vi "DeferPanelUpdate.vi"(8 "VI in":refnum<vi>, 10 "defer panel updates":bool, 11 "error in (no error)":errorcluster) -> (0 "VI out":refnum<vi>, 3 "error out":errorcluster)   [LabVIEW 2013]
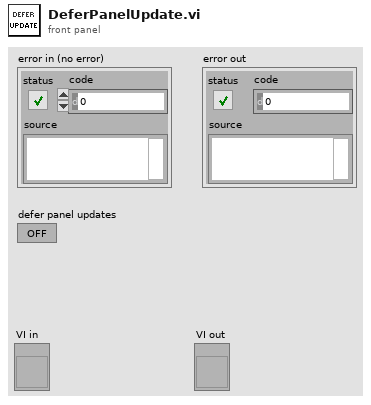
[diagram p1: front panel]
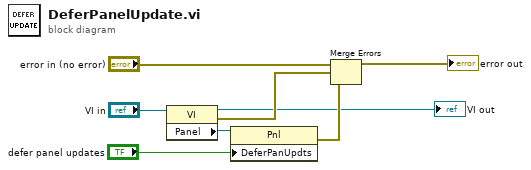
[diagram p0: block diagram]
diagram:
  n1 = property class="VI"(reference="VI in") -> (reference out=→"VI out":refnum<vi>, error out=w3:errorcluster, "Panel"=w4:refnum<vi>)  [unwired: 1 in]
  n2 = property class="Pnl"(reference=w4, "DeferPanUpdts"="defer panel updates") -> (error out=w2:errorcluster)  [unwired: 1 in, 1 out]
  n3 = Merge Errors("error in (no error)", w3, w2) -> (→"error out":errorcluster)
